vi "Unloop Timestamp.vi"(10 "Initialize?":bool, 11 "Time String":string) -> (3 "Corrected Time Stamp":timestamp)   [LabVIEW 2019, in "Muon Data Post-Processing.lvlib"]
uses:
  Muon Data Post-Processing.lvlib
panel:
  out "Offset Counter":i32
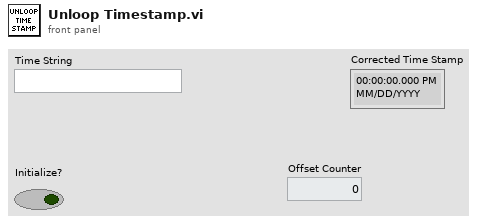
[diagram p1: front panel]
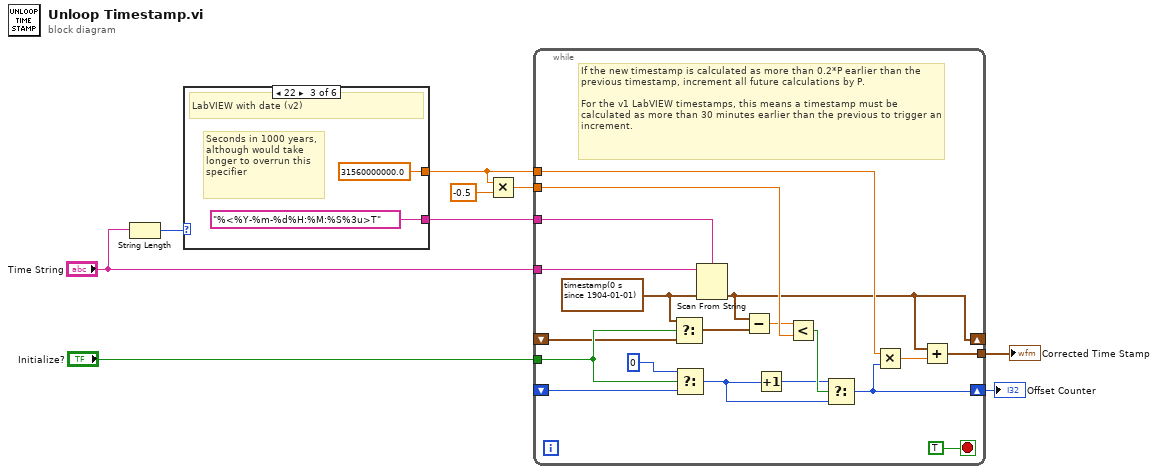
[diagram p0: block diagram]
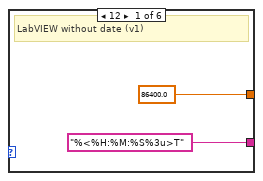
[diagram p2: hidden frame]
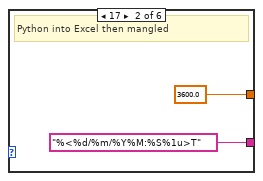
[diagram p3: hidden frame]
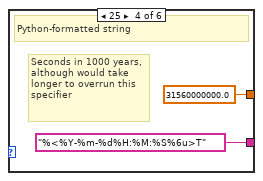
[diagram p4: hidden frame]
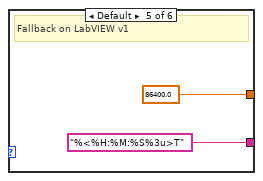
[diagram p5: hidden frame]
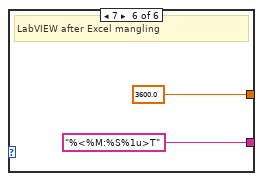
[diagram p6: hidden frame]
diagram:
  n1 = String Length(string="Time String") -> (length=w9:i32)
  n2 = case shown="22" w9 {
    tunnel: ["%<%H:%M:%S%3u>T" "%<%d/%m/%Y%M:%S%1u>T" "%<%Y-%m-%d%H:%M:%S%3u>T" "%<%Y-%m-%d%H:%M:%S%6u>T" "%<%H:%M:%S%3u>T" "%<%M:%S%1u>T"] -> w7
    tunnel: [86400.0 3600.0 31560000000.0 31560000000.0 86400.0 3600.0] -> w3
    frame 12 {
      # "LabVIEW without date (v1)"
    }
    frame 17 {
      # "Python into Excel then mangled"
    }
    frame 22 {
      # "Seconds in 1000 years, although would take longer to overrun this specifier"
      # "LabVIEW with date (v2)"
    }
    frame 25 {
      # "Seconds in 1000 years, although would take longer to overrun this specifier"
      # "Python-formatted string"
    }
    frame Default {
      # "Fallback on LabVIEW v1"
    }
    frame 7 {
      # "LabVIEW after Excel mangling"
    }
  }
  n3 = Multiply(x=w3, y=-0.5) -> (x*y=w2:dbl)
  n4 = while {
    tunnel: "Time String" -> [w38]
    tunnel: w7 -> [w37]
    tunnel: w3 -> [w25]
    shift-right: [w26] -> w4
    shift-left: _ -> [w36]
    tunnel: "Initialize?" -> [w34]
    shift-right: [w24] -> _
    shift-left: _ -> [w33]
    tunnel: w2 -> [w40]
    tunnel: [w22] -> w5
    stop <- TRUE stop-if-true
    w32 = timestamp(0 s since 1904-01-01) ("Time Stamp")
    # "If the new timestamp is calculated as more than 0.2*P earlier than the previous timestamp, increment all future calculations by P.\n\nFor the v1 LabVIEW timestamps, this means a timestamp must be calculated as more than 30 minutes earlier than the previous to trigger an increment."
    n5 = Select(t=w32, s=w34, f=w33) -> (s? t:f=w31:timestamp)
    n6 = Select(t=0, s=w34, f=w36) -> (s? t:f=w28:i32)
    n7 = Scan From String(format string=w37, input string=w38, default 1=w32) -> (output 1=w24:timestamp)  [unwired: 2 in, 3 out]
    n8 = Subtract(x=w24, y=w31) -> (x-y=w30:dbl)
    n9 = Increment(x=w28) -> (x+1=w27:i32)
    n10 = Less?(x=w30, y=w40) -> (x < y?=w29:bool)
    n11 = Select(t=w27, s=w29, f=w28) -> (s? t:f=w26:i32)
    n12 = Multiply(x=w25, y=w26) -> (x*y=w23:dbl)
    n13 = Add(x=w24, y=w23) -> (x+y=w22:timestamp)
  }
  "Corrected Time Stamp" <- w5
  "Offset Counter" <- w4
